vi "UpdatePropertyMethod.vi"(1 "VI":refnum<vi>, 2 "ClassItemRefIn":refnum<vi>, 3 "Property":string, 4 "PropertyObjectAttribute":bool, 5 "error IO":errorcluster, 6 "GetMethod":bool) -> (19 "error out":errorcluster)   [LabVIEW 2020, in "ClassWriterGOOP300.lvclass"]
uses:
  <resource>/Framework/Providers/Open_GDS/ClassProviders/Provider_EndevoGOOP300/ClassWriterGOOP300_class/ClassWriterGOOP300.lvclass
  <vilib>/Utility/miscctls.llb/LVPositionTypeDef.ctl
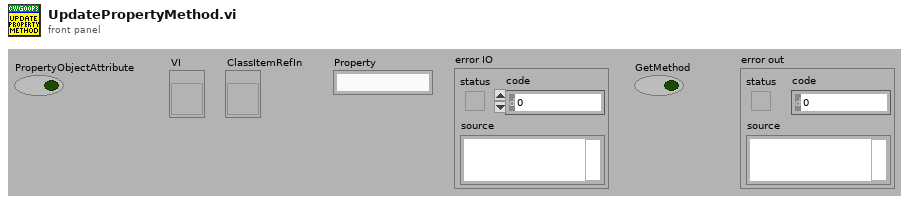
[diagram p1: front panel]
types:
  T1 = typedef "LVPositionTypeDef.ctl" = cluster{"Left":i32, "Top":i32}
  T2 = enum16{"Invalid Wire Rule", "Required", "Recommended", "Optional", "Dynamic Dispatch"}
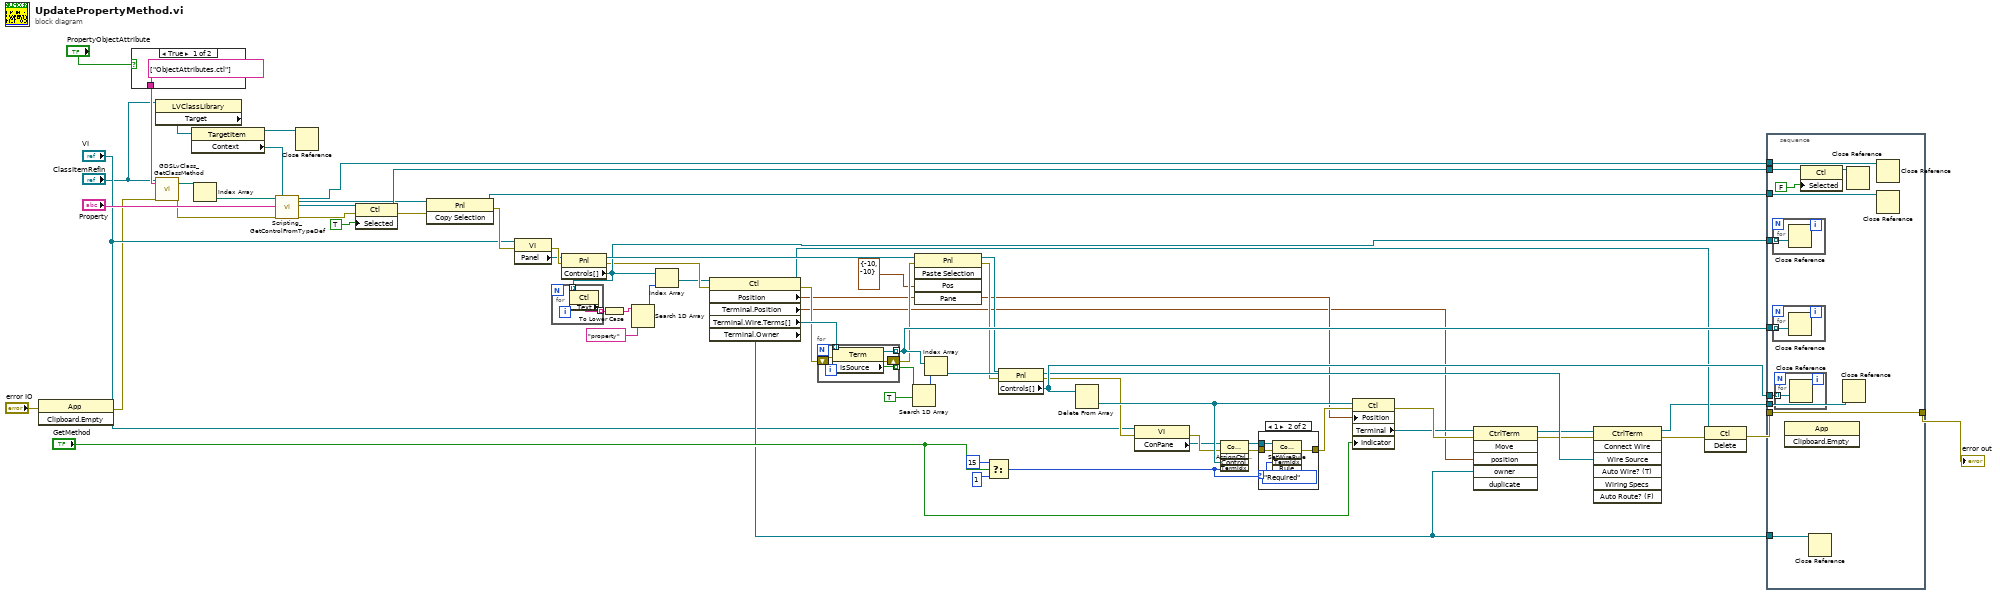
[diagram p0: block diagram]
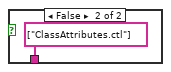
[diagram p3: hidden frame]
diagram:
  n1 = invoke class="App" method="Clipboard.Empty"(error in="error IO") -> (error out=w5:errorcluster)  [unwired: 2 in, 2 out]
  n2 = case shown="True" "PropertyObjectAttribute" {
    tunnel: [string[] ["ObjectAttributes.ctl"] ("VINames") string[] ["ClassAttributes.ctl"] ("VINames")] -> w29
    frame True {
    }
    frame False {
    }
  }
  n3 = property class="LVClassLibrary"(reference="ClassItemRefIn") -> ("Target"=w3:refnum<vi>)  [unwired: 1 in, 2 out]
  n4 = call <resource>:"GDSLvClass_GetClassMethod.vi"("Class Refnum In"="ClassItemRefIn", "VINames"=w29, "error in (no error)"=w5) -> ("ViPaths"=w30:path[], "error out"=w31:errorcluster)  [unwired: 13 in, 2 out]
  n5 = property class="TargetItem"(reference=w3) -> (reference out=w1:refnum<vi>, "Context"=w2:refnum<vi>)  [unwired: 1 in, 1 out]
  n6 = Index Array(array=w30) -> (element=w32:path)  [unwired: 1 in]
  n7 = call <resource>:"Scripting_GetControlFromTypeDef.vi"("TypeDefControl"=w32, "String"="Property", "error in"=w31, "AppRef"=w2) -> ("vi reference"=w8:refnum<vi>, "Panel"=w7:refnum<vi>, "ControlRef"=w35:refnum<vi>, "error out"=w37:errorcluster)  [unwired: 12 in]
  n8 = Close Reference(reference=w1) -> ()  [unwired: 1 in, 1 out]
  n9 = property class="Ctl"(reference=w35, error in=w37, "Selected"=TRUE) -> (reference out=w54:refnum<vi>, error out=w36:errorcluster)
  n10 = invoke class="Pnl" method="Copy Selection"(reference=w7, error in=w36) -> (reference out=w53:refnum<vi>, error out=w38:errorcluster)  [unwired: 1 in, 1 out]
  n11 = property class="VI"(reference="VI", error in=w38) -> (error out=w40:errorcluster, "Panel"=w39:refnum<vi>)  [unwired: 1 out]
  n12 = property class="Pnl"(reference=w39, error in=w40) -> (reference out=w59:refnum<vi>, error out=w45:errorcluster, "Controls[]"=w55:refnum<vi>[])
  n13 = for {
    tunnel: w55 -> [w71] mode=indexing
    tunnel: [w70] -> w41 mode=indexing
    n14 = property class="Ctl"(reference=w71) -> ("Label.Text"=w70:string)  [unwired: 1 in, 2 out]
  }
  n15 = To Lower Case(string=w41) -> (all lower case string=w58:string[])
  n16 = Search 1D Array(1D array=w58, element="property") -> (index of element=w43:i32)  [unwired: 1 in]
  n17 = Index Array(array=w55, index=w43) -> (element=w44:refnum<vi>)
  n18 = property class="Ctl"(reference=w44, error in=w45) -> (reference out=w23:refnum<vi>, error out=w27:errorcluster, "Position"=w18:T1, "Terminal.Position"=w12:T1, "Terminal.Wire.Terms[]"=w46:refnum<vi>[], "Terminal.Owner"=w10:refnum<vi>)
  n19 = for {
    tunnel: w46 -> [w76] mode=indexing
    tunnel: [w75] -> w47 mode=indexing
    tunnel: [w74] -> w56 mode=indexing
    shift-right: [w72] -> w26
    shift-left: w27 -> [w73]
    n20 = property class="Term"(reference=w76, error in=w73) -> (reference out=w74:refnum<vi>, error out=w72:errorcluster, "IsSource"=w75:bool)
  }
  n21 = Search 1D Array(1D array=w47, element=TRUE) -> (index of element=w49:i32)  [unwired: 1 in]
  n22 = invoke class="Pnl" method="Paste Selection"(reference=w59, error in=w26, "Pos"=T1 {"Left"=-10, "Top"=-10} ("Position")) -> (reference out=w50:refnum<vi>, error out=w22:errorcluster)  [unwired: 2 in, 3 out]
  n23 = Index Array(array=w56, index=w49) -> (element=w51:refnum<vi>)
  n24 = Select(t=u32 15 ("Terminal Index"), s="GetMethod", f=u32 1 ("Terminal Index")) -> (s? t:f=w67:u32)
  n25 = property class="Pnl"(reference=w50, error in=w22) -> (error out=w21:errorcluster, "Controls[]"=w57:refnum<vi>[])  [unwired: 1 out]
  n26 = Delete From Array(array=w57) -> (deleted portion=w62:refnum<vi>)  [unwired: 2 in, 1 out]
  n27 = property class="VI"(reference="VI", error in=w21) -> (error out=w61:errorcluster, "ConPane"=w60:refnum<vi>)  [unwired: 1 out]
  n28 = invoke class="ConPane" method="AssignCtrlToTerm"(reference=w60, error in=w61, "Control"=w62, "TermIdx"=w67) -> (reference out=w65:refnum<vi>, error out=w66:errorcluster)  [unwired: 1 in, 3 out]
  n29 = case shown="1" w67 {
    selector: w67 -> [_ w79]
    tunnel: w65 -> [_ w82]
    tunnel: w66 -> [w77 w81]
    tunnel: [w77 w78] -> w19
    frame 0, Default {
    }
    frame 1 {
      n30 = invoke class="ConPane" method="SetWireRule"(reference=w82, error in=w81, "TermIdx"=w79, "Rule"=T2."Required") -> (error out=w78:errorcluster)  [unwired: 1 in, 4 out]
    }
  }
  n31 = property class="Ctl"(reference=w62, error in=w19, "Position"=w18, "Indicator"="GetMethod") -> (error out=w15:errorcluster, "Terminal"=w14:refnum<vi>)  [unwired: 1 out]
  n32 = invoke class="CtrlTerm" method="Move"(reference=w14, error in=w15, "position"=w12, "owner"=w10) -> (reference out=w13:refnum<vi>, error out=w11:errorcluster)  [unwired: 2 in, 4 out]
  n33 = invoke class="CtrlTerm" method="Connect Wire"(reference=w13, error in=w11, "Wire Source"=w51) -> (reference out=w16:refnum<vi>, error out=w25:errorcluster)  [unwired: 4 in, 5 out]
  n34 = invoke class="Ctl" method="Delete"(reference=w23, error in=w25) -> (error out=w24:errorcluster)  [unwired: 1 in, 2 out]
  n35 = stacked-sequence {
    tunnel: w24 -> [w93]
    tunnel: [w93] -> w52
    tunnel: w8 -> [w92]
    tunnel: w53 -> [w91]
    tunnel: w54 -> [w84]
    tunnel: w55 -> [w90]
    tunnel: w56 -> [w89]
    tunnel: w57 -> [w88]
    tunnel: w16 -> [w87]
    tunnel: w10 -> [w86]
    frame #0 {
      n36 = for {
        tunnel: w90 -> [w96] mode=indexing
        n37 = Close Reference(reference=w96) -> ()  [unwired: 1 in, 1 out]
      }
      n38 = for {
        tunnel: w89 -> [w95] mode=indexing
        n39 = Close Reference(reference=w95) -> ()  [unwired: 1 in, 1 out]
      }
      n40 = for {
        tunnel: w88 -> [w94] mode=indexing
        n41 = Close Reference(reference=w94) -> ()  [unwired: 1 in, 1 out]
      }
      n42 = invoke class="App" method="Clipboard.Empty"() -> ()  [unwired: 3 in, 3 out]
      n43 = property class="Ctl"(reference=w84, "Selected"=FALSE) -> (reference out=w83:refnum<vi>)  [unwired: 1 in, 1 out]
      n44 = Close Reference(reference=w86) -> ()  [unwired: 1 in, 1 out]
      n45 = Close Reference(reference=w87) -> ()  [unwired: 1 in, 1 out]
      n46 = Close Reference(reference=w83) -> ()  [unwired: 1 in, 1 out]
      n47 = Close Reference(reference=w92) -> ()  [unwired: 1 in, 1 out]
      n48 = Close Reference(reference=w91) -> ()  [unwired: 1 in, 1 out]
    }
  }
  "error out" <- w52
